vi "Simple Serial.vi"() -> ()   [LabVIEW 2018]
doc: "This example performs a serial port write and a serial port read. The parameters set for the serial port must match the parameters of the connected instrument or device. The VISA Configure Serial Port VI sets the configuration parameters. The front panel displays the controls used to configure the basic parameters, such as baud rate, data bits, and parity. The VI passes the VISA resource name to other VIs that perform operations on that VISA resource. The VISA Write function sends a command to the serial device and the VISA Read function returns data based on the command. The VISA Close function then closes the reference to the serial device. It is important to close the reference; otherwise, further communication through that port might not be possible."
uses:
  Program Files (x86)/National Instruments/LabVIEW 2018/examples/Instrument IO/Serial/support/Serial - Settings.ctl
  <vilib>/Instr/_visa.llb/VISA Configure Serial Port (Instr).vi
panel:
  out "light intensity":u16
  out "red":u16
  out "green":u16
  out "blue":u16
  out "Button Sensor":bool
  out "accX 2":i16
  out "accY 2":i16
  out "accZ 2":i16
  out "ultrasonic distance (mm)":dbl
  out "B4":bool
  out "B3":bool
  out "B2":bool
  out "B1":bool
  out "temperature":dbl
  out "accZ":i16
  out "accY":i16
  out "accX":i16
  out "batteryVoltage":dbl
  out "corruptedTicks":u8
  in  "Init":bool
  out "sensros list":string[](array[string])
  in  "Sync":bool
  in  "stop":bool
  in  "Serial Settings":T1={"baud rate"=9600, "data bits"=8, "parity"=enum."None", "stop bits"=10, "flow control"=0} {"flow control" items=["None"=0, "XON/XOFF"=1, "RTS/CTS"=2, "DTR/DSR"=4]; "stop bits" items=["1.0"=10, "1.5"=15, "2.0"=20]; "data bits" min=5 max=8 step=1; "baud rate" items=["75"=75, "110"=110, "134"=134, "150"=150, "300"=300, "600"=600, "1200"=1200, "1800"=1800, "2400"=2400, "4800"=4800, "7200"=7200, "9600"=9600, "14400"=14400, "19200"=19200, "28800"=28800, "38400"=38400, "56000"=56000, "57600"=57600, "115200"=115200, "128000"=128000, "230400"=230400]}
  out "bytes read":u32
  out "Response":string
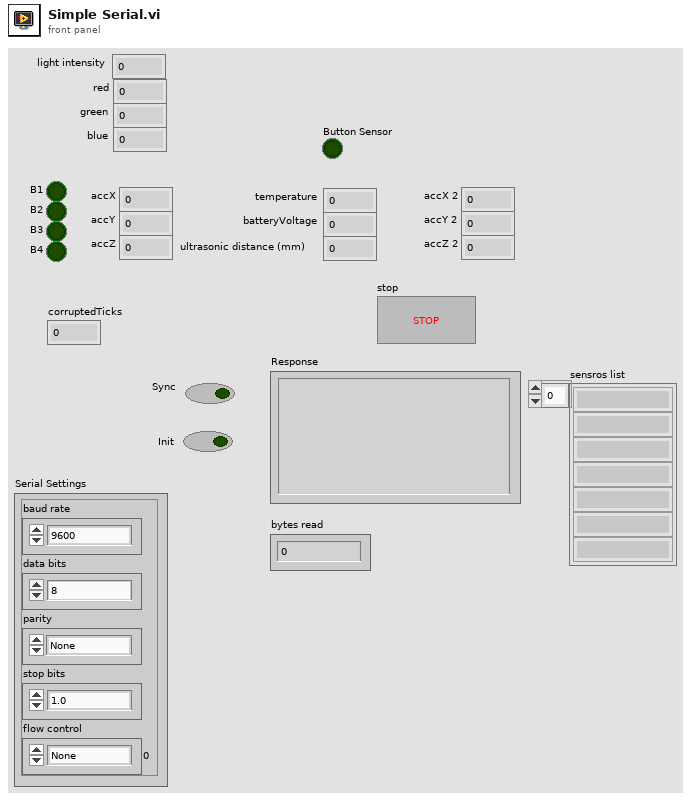
[diagram p1: front panel]
types:
  T1 = typedef "Serial - Settings.ctl" = cluster{"baud rate":u32, "data bits":u16, "parity":enum16{"None", "Odd", "Even", "Mark", "Space"}, "stop bits":u16, "flow control":u16}
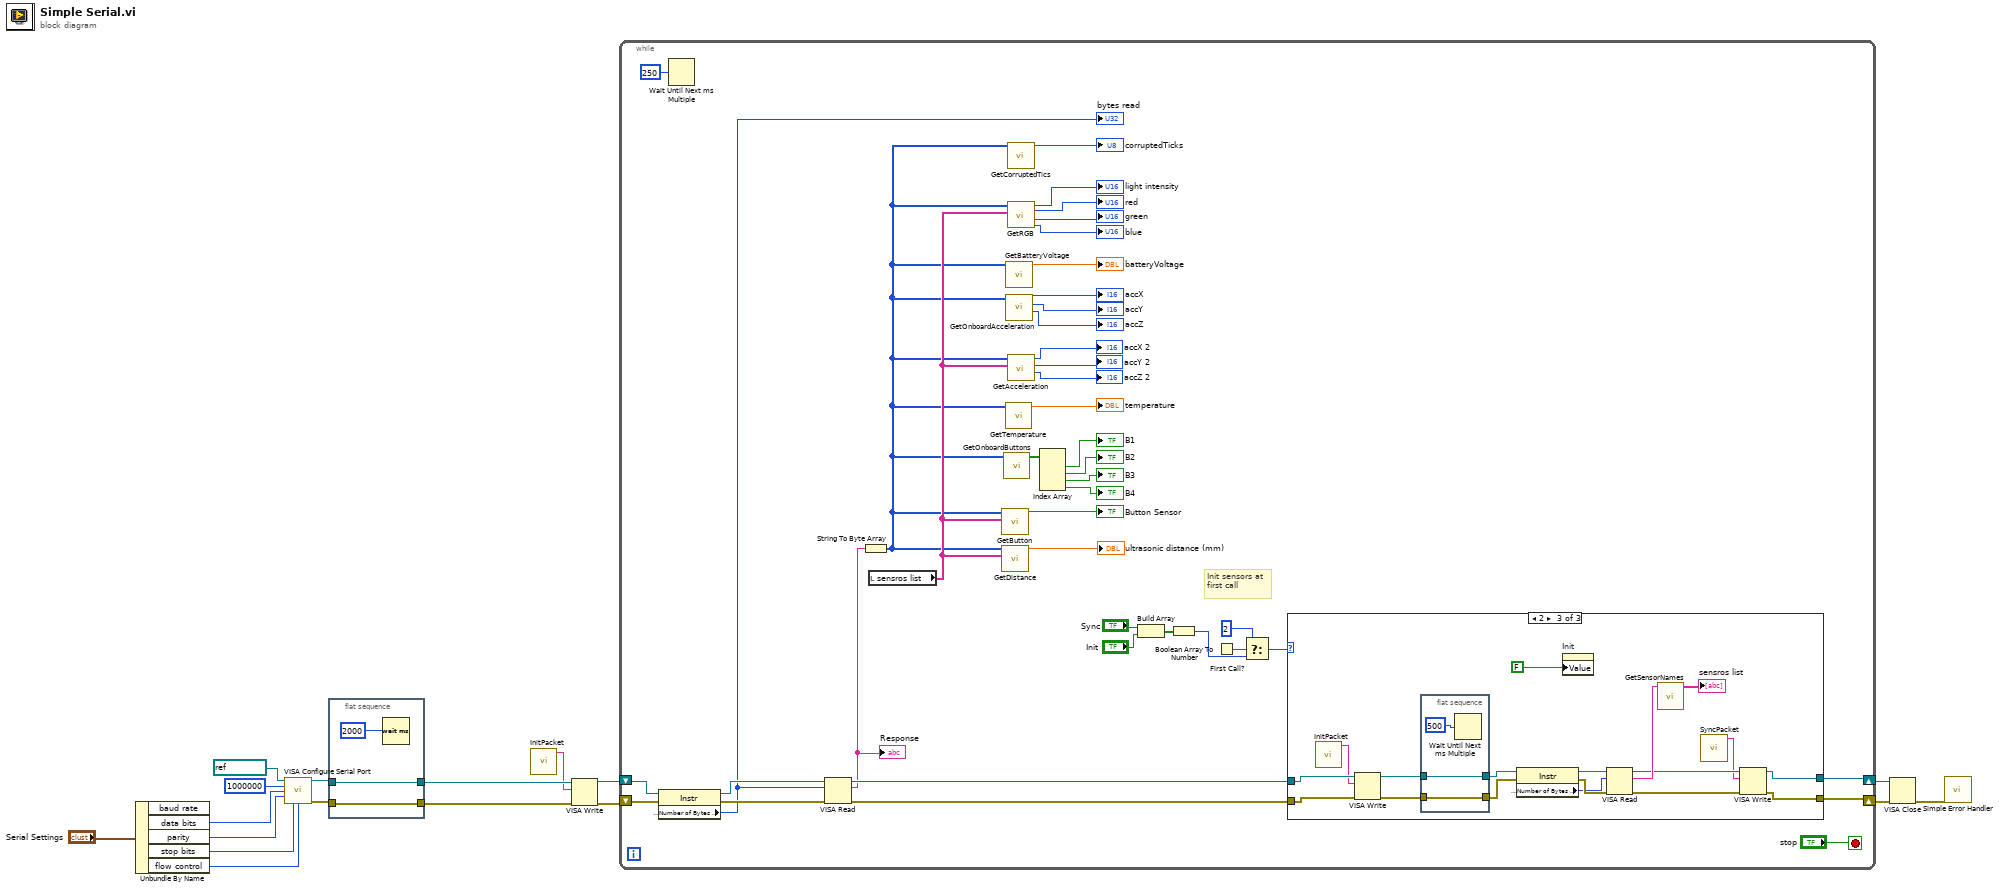
[diagram p0: block diagram]
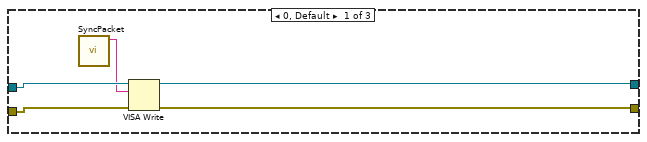
[diagram p2: hidden frame]
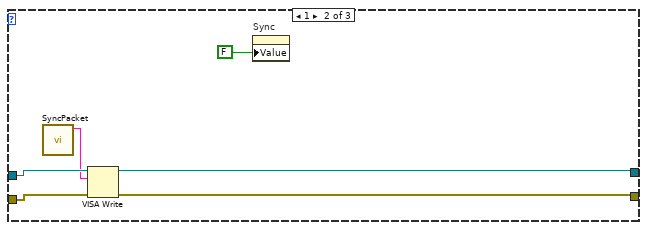
[diagram p3: hidden frame]
diagram:
  n1 = Unbundle By Name("Serial Settings") -> ("data bits"=w11:u16, "parity"=w10:enum16{"None", "Odd", "Even", "Mark", "Space"}, "stop bits"=w9:u16, "flow control"=w8:u16)  [unwired: 1 out]
  n2 = call-poly "VISA Configure Serial Port"("VISA resource name"=refnum<visa-resource-name> "COM8", "baud rate (9600)"=u32 1000000, "data bits (8)"=w11, "parity (0:none)"=w10, "stop bits (10: 1 bit)"=w9, "flow control (0:none)"=w8) -> ("VISA resource name out"=w16:refnum<visa-resource-name>, "error out"=w2:errorcluster)  [unwired: 3 in, 5 out]
  n3 = flat-sequence {
    tunnel: w2 -> [w20]
    tunnel: [w20] -> w3
    tunnel: w16 -> [w19]
    tunnel: [w19] -> w4
    frame #0 {
      n4 = Wait (ms)(milliseconds to wait=u32 2000 ("delay before read (ms)")) -> ()  [unwired: 1 out]
    }
  }
  n5 = call "InitPacket.vi"() -> ("string"=w1:string)  [unwired: 11 in]
  n6 = VISA Write(VISA resource name=w4, write buffer=w1, error in (no error)=w3) -> (VISA resource name out=w5:refnum<visa-resource-name>, error out=w6:errorcluster)  [unwired: 1 out]
  n7 = while {
    shift-right: [w49] -> w15
    shift-left: w6 -> [w61]
    shift-right: [w50] -> w14
    shift-left: w5 -> [w60]
    stop <- "stop" stop-if-true
    # "Init sensors at first call"
    n8 = property class="Instr"(reference=w60, error in=w61) -> (reference out=w59:refnum<visa-resource-name>, error out=w58:errorcluster, "Serial Settings:Number of Bytes at Serial Port"=w48:u32)
    "bytes read" <- w48
    n9 = Wait Until Next ms Multiple(millisecond multiple=u32 250) -> ()  [unwired: 1 out]
    n10 = VISA Read(VISA resource name=w59, byte count=w48, error in (no error)=w58) -> (VISA resource name out=w54:refnum<visa-resource-name>, read buffer=w36:string, error out=w55:errorcluster)  [unwired: 1 out]
    "Response" <- w36
    n11 = String To Byte Array(string=w36) -> (unsigned byte array=w25:u8[])
    n12 = local read "sensros list"() -> (w26:string[])
    n13 = call "GetButton.vi"("sensors list"=w26, "packet in"=w25) -> ("button state"=→"Button Sensor":bool)  [unwired: 9 in]
    n14 = call "GetDistance.vi"("sensors list"=w26, "packet in"=w25) -> ("distance (mm)"=→"ultrasonic distance (mm)":dbl)  [unwired: 9 in]
    n15 = call "GetOnboardButtons.vi"("packet in"=w25) -> ("onboard buttons state"=w32:bool[])  [unwired: 10 in]
    n16 = call "GetTemperature.vi"("packet in"=w25) -> ("temperature (degC)"=→"temperature":dbl)  [unwired: 10 in]
    n17 = call "GetBatteryVoltage.vi"("packet in"=w25) -> ("battery voltage (V)"=→"batteryVoltage":dbl)  [unwired: 10 in]
    n18 = call "GetOnboardAcceleration.vi"("packet in"=w25) -> ("accZ"=→"accZ":i16, "accY"=→"accY":i16, "accX"=→"accX":i16)  [unwired: 8 in]
    n19 = call "GetCorruptedTics.vi"("packet in"=w25) -> ("corrupted ticks"=→"corruptedTicks":u8)  [unwired: 10 in]
    n20 = call "GetRGB.vi"("sensors list"=w26, "packet in"=w25) -> ("blue"=→"blue":u16, "green"=→"green":u16, "red"=→"red":u16, "light intensity"=→"light intensity":u16)  [unwired: 6 in]
    n21 = call "GetAcceleration.vi"("sensors list"=w26, "packet in"=w25) -> ("accZ"=→"accZ 2":i16, "accY"=→"accY 2":i16, "accX"=→"accX 2":i16)  [unwired: 7 in]
    n22 = Index Array(array=w32) -> (element #1=→"B1":bool, element #2=→"B2":bool, element #3=→"B3":bool, element #4=→"B4":bool)  [unwired: 4 in]
    n23 = Build Array("Sync", "Init") -> (w51:bool[])
    n24 = Boolean Array To Number(Boolean array=w51) -> (number=w22:u32)
    n25 = First Call?() -> (First Call?: T/F=w24:bool)
    n26 = Select(t=u32 2, s=w24, f=w22) -> (s? t:f=w23:u32)
    n27 = case shown="2" w23 {
      tunnel: w55 -> [w64 w71 w90]
      tunnel: w54 -> [w63 w70 w89]
      tunnel: [w66 w69 w75] -> w49
      tunnel: [w65 w68 w76] -> w50
      frame 0, Default {
        n28 = call "SyncPacket.vi"() -> ("sync packet"=w62:string)  [unwired: 11 in]
        n29 = VISA Write(VISA resource name=w63, write buffer=w62, error in (no error)=w64) -> (VISA resource name out=w65:refnum<visa-resource-name>, error out=w66:errorcluster)  [unwired: 1 out]
      }
      frame 1 {
        n30 = call "SyncPacket.vi"() -> ("sync packet"=w67:string)  [unwired: 11 in]
        n31 = VISA Write(VISA resource name=w70, write buffer=w67, error in (no error)=w71) -> (VISA resource name out=w68:refnum<visa-resource-name>, error out=w69:errorcluster)  [unwired: 1 out]
        n32 = property on="Sync" class="Bool (strict)"("Value"=FALSE ("Boolean")) -> ()  [unwired: 2 in, 2 out]
      }
      frame 2 {
        n33 = call "InitPacket.vi"() -> ("string"=w74:string)  [unwired: 11 in]
        n34 = VISA Write(VISA resource name=w89, write buffer=w74, error in (no error)=w90) -> (VISA resource name out=w86:refnum<visa-resource-name>, error out=w87:errorcluster)  [unwired: 1 out]
        n35 = flat-sequence {
          tunnel: [w92] -> w84
          tunnel: w87 -> [w92]
          tunnel: [w91] -> w83
          tunnel: w86 -> [w91]
          frame #0 {
            n36 = Wait Until Next ms Multiple(millisecond multiple=u32 500) -> ()  [unwired: 1 out]
          }
        }
        n37 = property class="Instr"(reference=w83, error in=w84) -> (reference out=w80:refnum<visa-resource-name>, error out=w82:errorcluster, "Serial Settings:Number of Bytes at Serial Port"=w81:u32)
        n38 = property on="Init" class="Bool (strict)"("Value"=FALSE ("Init")) -> ()  [unwired: 2 in, 2 out]
        n39 = VISA Read(VISA resource name=w80, byte count=w81, error in (no error)=w82) -> (VISA resource name out=w77:refnum<visa-resource-name>, read buffer=w79:string, error out=w78:errorcluster)  [unwired: 1 out]
        n40 = call "GetSensorNames.vi"("read buffer"=w79) -> ("sensors names"=→"sensros list":string[])  [unwired: 10 in]
        n41 = call "SyncPacket.vi"() -> ("sync packet"=w73:string)  [unwired: 11 in]
        n42 = VISA Write(VISA resource name=w77, write buffer=w73, error in (no error)=w78) -> (VISA resource name out=w76:refnum<visa-resource-name>, error out=w75:errorcluster)  [unwired: 1 out]
      }
    }
  }
  n43 = VISA Close(VISA resource name=w14, error in (no error)=w15) -> (error out=w13:errorcluster)
  n44 = call <vilib>:"Simple Error Handler.vi"("error in (no error)"=w13) -> ()  [unwired: 1 in, 8 out]
